vi "DistancesFromOrigin.vi"(8 "error in (no error)":errorcluster, 10 "Image Dst":T1, 11 "Image Src":T1) -> (0 "error out":errorcluster, 2 "Image Out":T1, 3 "Array":string[](array[string]))   [LabVIEW 2020]
doc: "Disegna un overlay con la distanza dall'origine."
uses:
  <vilib>/vision/Image Controls.llb/IMAQ Image.ctl
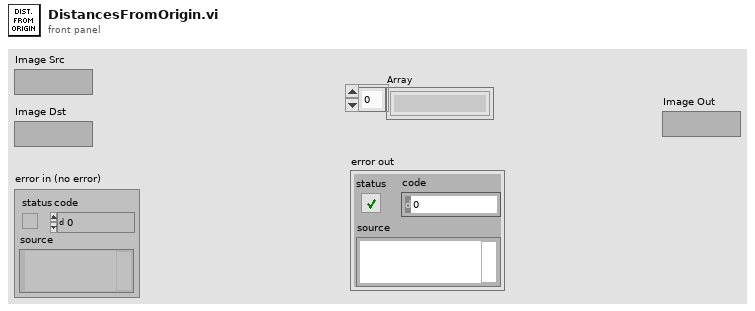
[diagram p1: front panel]
types:
  T1 = typedef "IMAQ Image.ctl" = refnum<image>
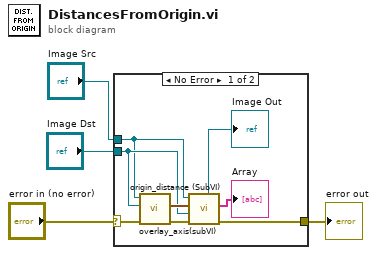
[diagram p0: block diagram]
diagram:
  n1 = case shown="No Error" "error in (no error)" {
    selector: "error in (no error)" -> [w8 w13]
    tunnel: "Image Src" -> [w5 _]
    tunnel: [w12 w13] -> w2
    tunnel: "Image Dst" -> [w7 _]
    frame No Error {
      n2 = call "overlay_axis(subVI).vi"("error in (no error)"=w8, "image dst"=w7, "image src"=w5) -> ("error out"=w9:errorcluster, "Origin Pixel"=w10:cluster{"X":sgl, "Y":sgl})  [unwired: 6 in, 1 out]
      n3 = call "origin_distance (SubVI).vi"("error in (no error)"=w9, "Image Dst"=w7, "Origin Pixel"=w10, "Image Src"=w5) -> ("error out"=w12:errorcluster, "Array"=→"Array":string[], "Image Out"=→"Image Out":T1)  [unwired: 3 in, 2 out]
    }
    frame Error {
    }
  }
  "error out" <- w2
